vi "Pre Launch Init.vi"(11 "Flex  Dialog (Actor) in":refnum<class "Flex Dialog (Actor).lvclass">) -> (0 "error out":errorcluster, 3 "Flex  Dialog (Actor) out":refnum<class "Flex Dialog (Actor).lvclass">)   [LabVIEW 2016, in "Flex UI Dialog (Actor).lvlib" / "Flex Dialog (Actor).lvclass"]
doc: "(<B>Filename</B>: Actor Framework.lvlib:Actor.lvclass:Pre Launch Init.vi)\n\nDefines behavior that occurs after the Launch Nested Actor method is invoked but before the actor's Actor Core method begins running.\n\nBy default, this method does nothing. A descendant class may override it to define behavior."
uses:
  Flex Dialog (Actor).lvclass
  Flex Dialog (Actor).lvclass/Flex Dialog (Actor).ctl
  Flex UI (Actor)/Flex UI (Actor).lvclass
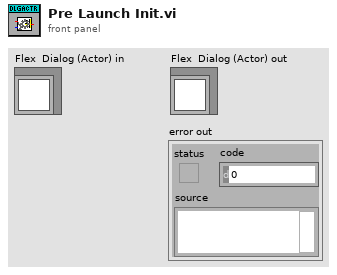
[diagram p1: front panel]
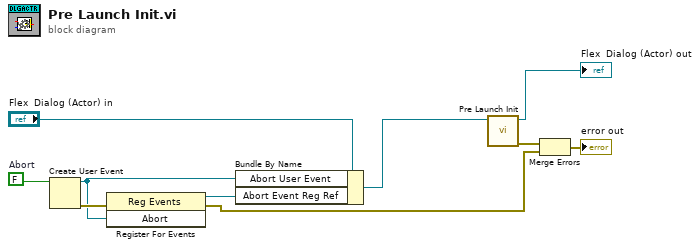
[diagram p0: block diagram]
diagram:
  w8 = FALSE  # Abort
  n1 = Create User Event(user event datatype=w8) -> (user event=w6:refnum<user-event>, error out=w7:errorcluster)  [unwired: 1 in]
  n2 = register-events(error in=w7, w6) -> (reference out=w5:refnum<event-registration>, error out=w2:errorcluster)  [unwired: 1 in]
  n3 = Bundle By Name(cluster="Flex  Dialog (Actor) in", "Abort User Event"=w6, "Abort Event Reg Ref"=w5) -> (w1:refnum<class "Flex Dialog (Actor).lvclass">)
  n4 = call-parent "Pre Launch Init.vi"("_Parent Actor Template in"=w1) -> ("error out"=w10:errorcluster, "_Parent Actor Template out"=→"Flex  Dialog (Actor) out":refnum<class "Flex Dialog (Actor).lvclass">)  [unwired: 9 in]
  n5 = Merge Errors(w10, w2) -> (→"error out":errorcluster)
